vi "变体转U8数组.vi"(8 "错误输入（无错误）":errorcluster, 11 "Value":variant) -> (0 "error out":errorcluster, 3 "U8数组":u8[](array[numeric]))   [LabVIEW 2022 SP3, in "斯坦道CODcr.lvlib"]
uses:
  <vilib>/Utility/Data Type/NI_Data Type.lvlib
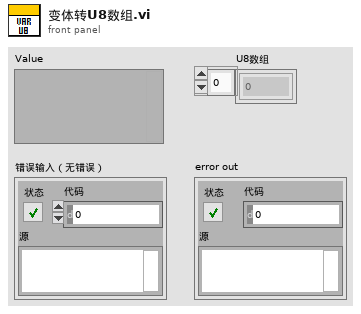
[diagram p1: front panel]
types:
  T1 = typedef "NI_Data Type.lvlib/Data Type.ctl" = enum8{"Invalid Type", "Void", "I8", "I16", "I32", "I64", "U8", "U16", "U32", "U64", "Single Float", "Double Float", "Extended Float", "Single Complex", "Double Complex", "Extended Complex", "Enum U8", "Enum U16", "Enum U32", "Enum U64", "Single Float With Unit", "Double Float With Unit", "Extended Float With Unit", "Single Complex with Unit", "Double Complex with Unit", "Extended Complex with Unit", "Boolean", "String", "Path", "Picture", "Tag", "Array", "Cluster", "Variant", "LV Variant", "Waveform", "Timestamp", "Digital Waveform", "Digital Data", "ExpressData", "Refnum", "External Data", "VI", "Poly VI", "LabVIEW Class Instance", "Fixed Point", "Set Collection", "Map Collection"}
  T2 = cluster{"标准值":sgl, "吸光值":sgl, "启用":bool, "数据时间":timestamp}
  T3 = typedef "LVDateTimeRec.ctl" = cluster{"秒数的小数部分":dbl, "秒":i32, "分":i32, "时":i32, "日":i32, "月":i32, "年":i32, "天数（周）":i32, "天数（年）":i32, "DST":i32}
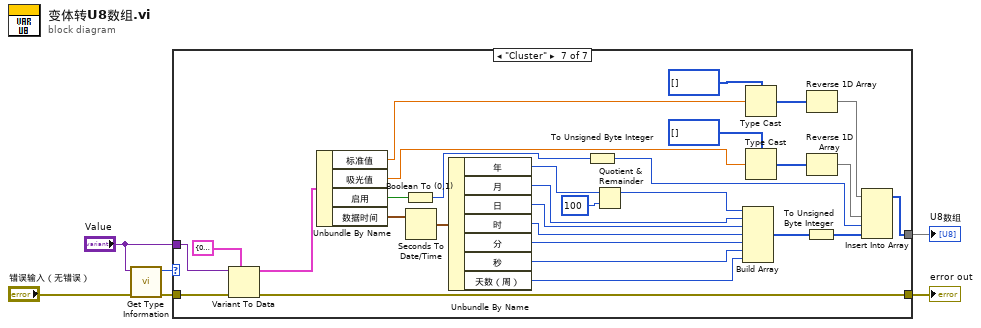
[diagram p0: block diagram]
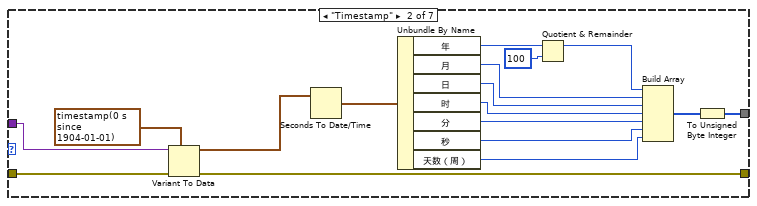
[diagram p3: hidden frame]
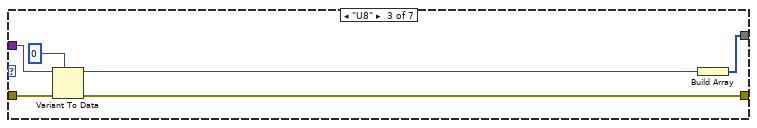
[diagram p4: hidden frame]
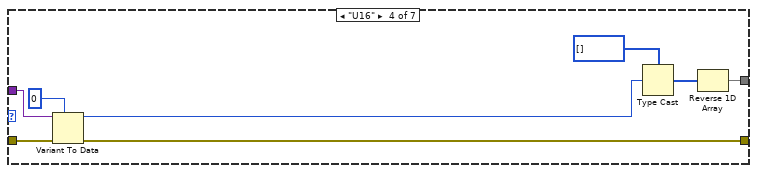
[diagram p5: hidden frame]
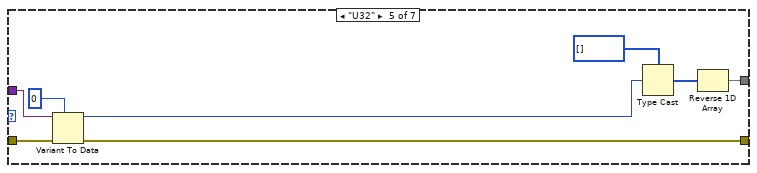
[diagram p6: hidden frame]
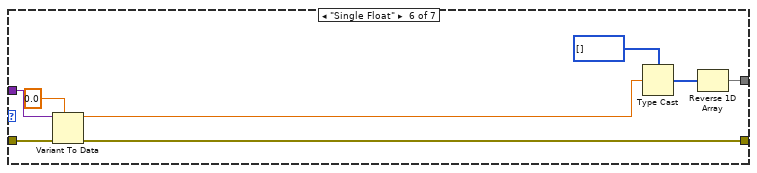
[diagram p7: hidden frame]
diagram:
  n1 = call <vilib>:"Get Type Information.vi"("error in (no error)"="错误输入（无错误）", "variant"="Value") -> ("error out"=w3:errorcluster, "type"=w4:T1)  [unwired: 5 in, 3 out]
  n2 = case shown="\"Cluster\"" w4 {
    tunnel: [_ w10 w30 w36 w44 w52 w70] -> w1
    tunnel: "Value" -> [_ w13 w28 w35 w43 w51 w84]
    tunnel: w3 -> [w7 w9 w26 w32 w40 w48 w56]
    tunnel: [w7 w8 w25 w31 w39 w47 w55] -> w2
    frame "Invalid Type", Default {
    }
    frame "Timestamp" {
      n3 = Variant To Data(error in=w9, type=timestamp(0 s since 1904-01-01) ("时间标识"), Variant=w13) -> (data=w11:timestamp, error out=w8:errorcluster)
      n4 = Seconds To Date/Time(time stamp (now)=w11) -> (date time rec=w24:T3)  [unwired: 1 in]
      n5 = Unbundle By Name(w24) -> ("年"=w23:i32, "月"=w20:i32, "日"=w19:i32, "时"=w18:i32, "分"=w17:i32, "秒"=w16:i32, "天数（周）"=w15:i32)
      n6 = Quotient & Remainder(x=w23, y=100) -> (x-y*floor(x/y)=w21:i32)  [unwired: 1 out]
      n7 = Build Array(w21, w20, w19, w18, w17, w16, w15) -> (w14:i32[])
      n8 = To Unsigned Byte Integer(number=w14) -> (unsigned 8bit integer=w10:u8[])
    }
    frame "U8" {
      n9 = Variant To Data(error in=w26, type=u8 0, Variant=w28) -> (data=w27:u8, error out=w25:errorcluster)
      n10 = Build Array(w27) -> (w30:u8[])
    }
    frame "U16" {
      n11 = Variant To Data(error in=w32, type=u16 0, Variant=w35) -> (data=w33:u16, error out=w31:errorcluster)
      n12 = Type Cast(type=u8[] [], x=w33) -> (*(type *) &x=w38:u8[])
      n13 = Reverse 1D Array(array=w38) -> (reversed array=w36:u8[])
    }
    frame "U32" {
      n14 = Variant To Data(error in=w40, type=u32 0, Variant=w43) -> (data=w41:u32, error out=w39:errorcluster)
      n15 = Type Cast(type=u8[] [], x=w41) -> (*(type *) &x=w46:u8[])
      n16 = Reverse 1D Array(array=w46) -> (reversed array=w44:u8[])
    }
    frame "Single Float" {
      n17 = Variant To Data(error in=w48, type=sgl 0.0, Variant=w51) -> (data=w49:sgl, error out=w47:errorcluster)
      n18 = Type Cast(type=u8[] [], x=w49) -> (*(type *) &x=w54:u8[])
      n19 = Reverse 1D Array(array=w54) -> (reversed array=w52:u8[])
    }
    frame "Cluster" {
      n20 = Variant To Data(error in=w56, type=T2 {"标准值"=0.0, "吸光值"=0.0, "启用"=FALSE, "数据时间"=timestamp(0 s since 1904-01-01)} ("校准值一"), Variant=w84) -> (data=w82:T2, error out=w55:errorcluster)
      n21 = Unbundle By Name(w82) -> ("标准值"=w79:sgl, "吸光值"=w76:sgl, "启用"=w75:bool, "数据时间"=w57:timestamp)
      n22 = Boolean To (0,1)(Boolean=w75) -> (0, 1=w74:i16)
      n23 = Seconds To Date/Time(time stamp (now)=w57) -> (date time rec=w69:T3)  [unwired: 1 in]
      n24 = Unbundle By Name(w69) -> ("年"=w68:i32, "月"=w65:i32, "日"=w64:i32, "时"=w63:i32, "分"=w62:i32, "秒"=w61:i32, "天数（周）"=w60:i32)
      n25 = To Unsigned Byte Integer(number=w74) -> (unsigned 8bit integer=w71:u8)
      n26 = Quotient & Remainder(x=w68, y=100) -> (x-y*floor(x/y)=w66:i32)  [unwired: 1 out]
      n27 = Build Array(w66, w65, w64, w63, w62, w61, w60) -> (w59:i32[])
      n28 = Type Cast(type=u8[] [], x=w79) -> (*(type *) &x=w81:u8[])
      n29 = Type Cast(type=u8[] [], x=w76) -> (*(type *) &x=w78:u8[])
      n30 = To Unsigned Byte Integer(number=w59) -> (unsigned 8bit integer=w58:u8[])
      n31 = Reverse 1D Array(array=w81) -> (reversed array=w73:u8[])
      n32 = Reverse 1D Array(array=w78) -> (reversed array=w72:u8[])
      n33 = Insert Into Array(array=w73, new element #1=w72, new element #2=w71, new element #3=w58) -> (w70:u8[])  [unwired: 1 in]
    }
  }
  "U8数组" <- w1
  "error out" <- w2
